vi "Parse Unregister Message.vi"(0 "State":string, 1 "Module Name":string, 5 "Args":string) -> (4 "Target":string, 6 "Source":string, 8 "Status":string, 10 "Api":string, 15 "Target Specified?":bool)   [LabVIEW 2017, in "Communicable State Machine.lvlib"]
doc: "### Parse Unregister Message.vi\n\n-- <b>Controls</b> --\n- <b>state</b>:\n- <b>Module Name </b>:\n- <b>args</b>:\n\n-- <b>Indicators</b> --\n- <b>target</b>:\n- <b>source</b>:\n- <b>status</b>:\n- <b>api</b>:"
uses:
  Communicable State Machine.lvlib
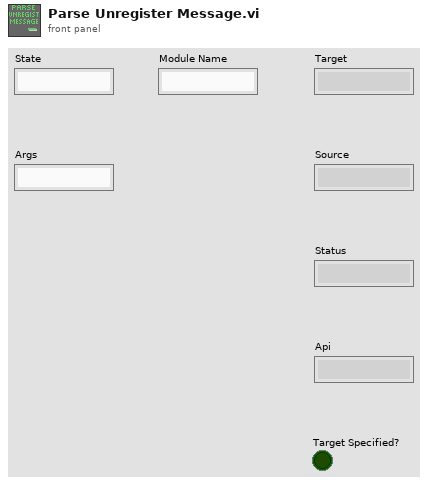
[diagram p1: front panel]
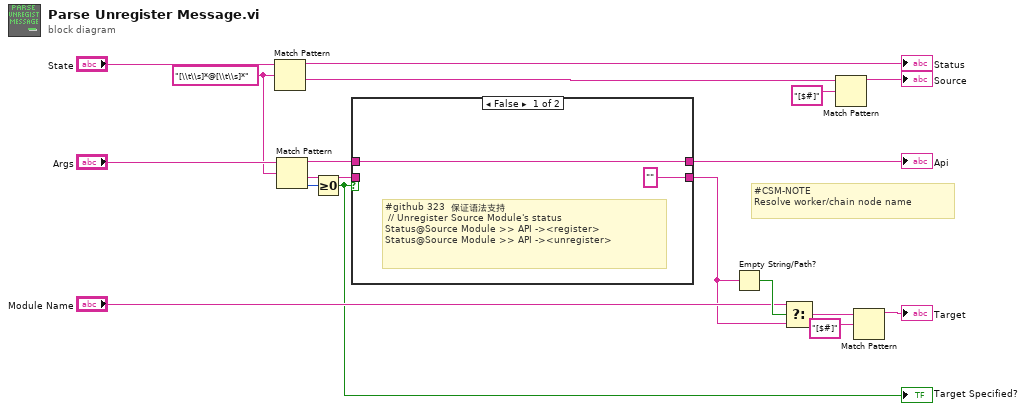
[diagram p0: block diagram]
diagram:
  w16 = "[\\t\\s]*@[\\t\\s]*" ("regular expression")
  # "#CSM-NOTE\nResolve worker/chain node name"
  n1 = Match Pattern(string="State", regular expression=w16) -> (before substring=→"Status":string, after substring=w14:string)  [unwired: 1 in, 2 out]
  n2 = Match Pattern(string="Args", regular expression=w16) -> (before substring=w10:string, after substring=w13:string, offset past match=w12:i32)  [unwired: 1 in, 1 out]
  n3 = Greater Or Equal To 0?(x=w12) -> (x >= 0?=w6:bool)
  "Target Specified?" <- w6
  n4 = case shown="False" w6 {
    tunnel: w13 -> [_ w22]
    tunnel: ["" ("args") w22] -> w7
    tunnel: [w20 w21] -> w11
    tunnel: w10 -> [w20 w21]
    frame False {
      # "#github 323  保证语法支持\n // Unregister Source Module's status\nStatus@Source Module >> API -><register>\nStatus@Source Module >> API -><unregister>"
    }
    frame True {
    }
  }
  "Api" <- w11
  n5 = Empty String/Path?(string/path=w7) -> (empty?=w9:bool)
  n6 = Select(t="Module Name", s=w9, f=w7) -> (s? t:f=w5:string)
  n7 = Match Pattern(string=w14, regular expression="[$#]") -> (before substring=→"Source":string)  [unwired: 1 in, 3 out]
  n8 = Match Pattern(string=w5, regular expression="[$#]") -> (before substring=→"Target":string)  [unwired: 1 in, 3 out]
